vi "MC5e Validate Unit Selection.vi"(11 "Value":i32) -> (2 "Is Valid":bool, 3 "Disabled":T1(ring))   [LabVIEW 2020]
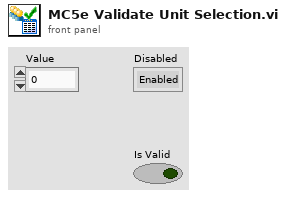
[diagram p1: front panel]
types:
  T1 = enum8{"Enabled", "Disabled", "Disabled and Grayed Out"}
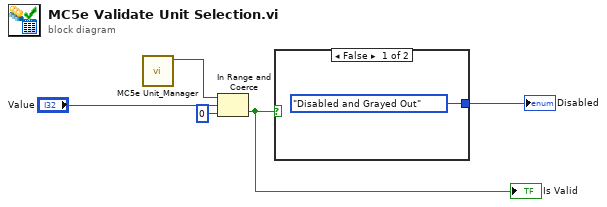
[diagram p0: block diagram]
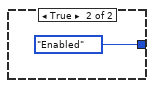
[diagram p2: hidden frame]
diagram:
  n1 = call "MC5e Unit_Manager.vi"() -> ("set size"=w1:i32)  [unwired: 8 in, 3 out]
  n2 = In Range and Coerce(upper limit=w1, x="Value", lower limit=0) -> (In Range?=w5:bool)  [unwired: 1 out]
  "Is Valid" <- w5
  n3 = case shown="False" w5 {
    tunnel: [T1."Disabled and Grayed Out" ("Disabled") T1."Enabled" ("Disabled")] -> w3
    frame False {
    }
    frame True {
    }
  }
  "Disabled" <- w3
